vi "Destroy User Events.vi"(11 "UI Template in":refnum<class "Nested.lvclass">) -> (3 "UI Template out":refnum<class "Nested.lvclass">)   [LabVIEW 2025, in "Nested.lvlib" / "Nested.lvclass"]
uses:
  Nested.lvclass
  Nested.lvclass/Nested.ctl
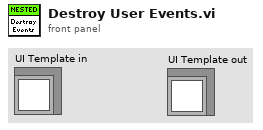
[diagram p1: front panel]
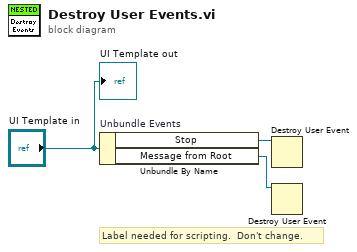
[diagram p0: block diagram]
diagram:
  # "Label needed for scripting.  Don't change."
  n1 = Unbundle By Name "Unbundle Events"("UI Template in") -> ("Stop"=w2:refnum<user-event>, "Message from Root"=w1:refnum<user-event>)
  n2 = Destroy User Event(user event=w2) -> ()  [unwired: 1 in, 1 out]
  n3 = Destroy User Event(user event=w1) -> ()  [unwired: 1 in, 1 out]
  "UI Template out" <- "UI Template in"
